vi "__Update Local List.vi"(8 "error in (no error)":errorcluster, 10 "Path to list":path, 11 "FileManager Ctl Refs in":T1) -> (0 "error out":errorcluster, 3 "FileManager Ctl Refs out":T1)   [LabVIEW 2011]
doc: "Lists the files and folders that reside under the specified path on the local system and updates the Local list with the items."
uses:
  __File manager Data type.ctl
  <vilib>/Utility/miscctls.llb/LVRowAndColumnUnsignedTypeDef.ctl
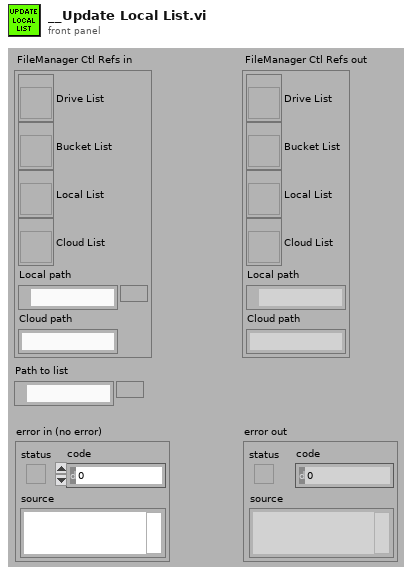
[diagram p1: front panel]
types:
  T1 = typedef "__File manager Data type.ctl" = cluster{"Drive List":refnum<vi>, "Bucket List":refnum<vi>, "Local List":refnum<vi>, "Cloud List":refnum<vi>, "Local path":path, "Cloud path":string}
  T2 = typedef "LVRowAndColumnUnsignedTypeDef.ctl" = cluster{"Row":u32, "Column":u32}
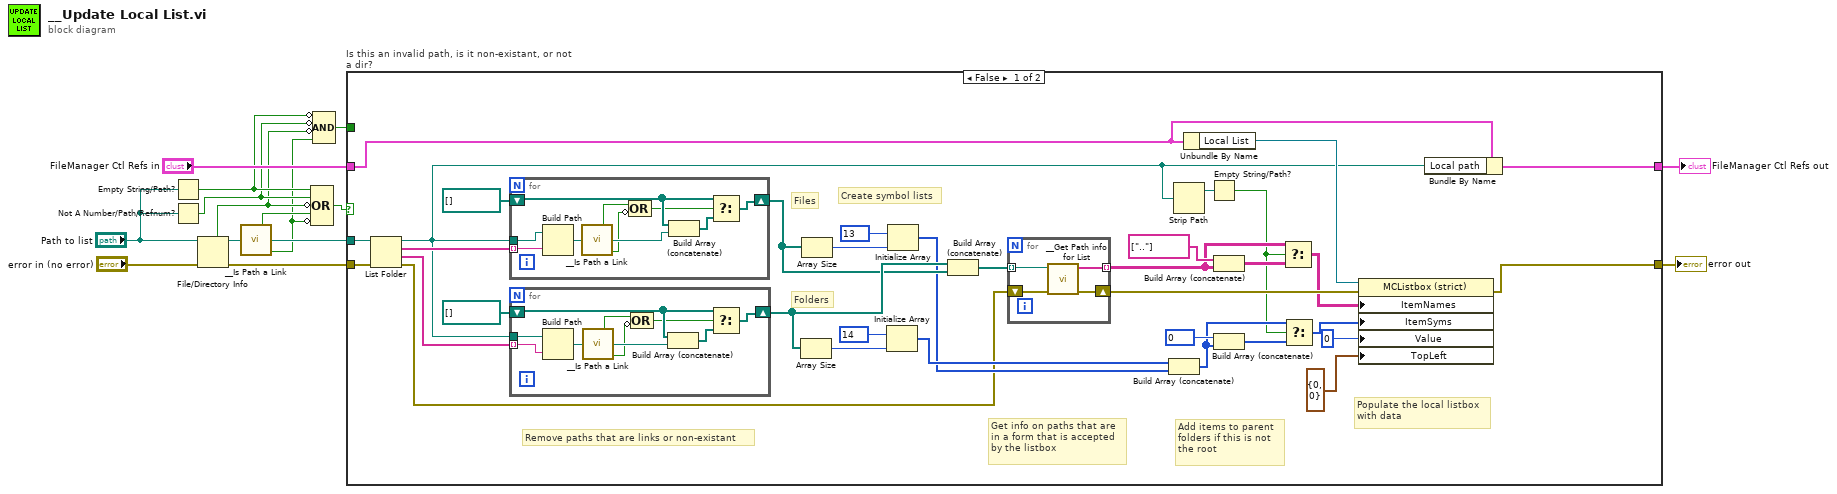
[diagram p0: block diagram]
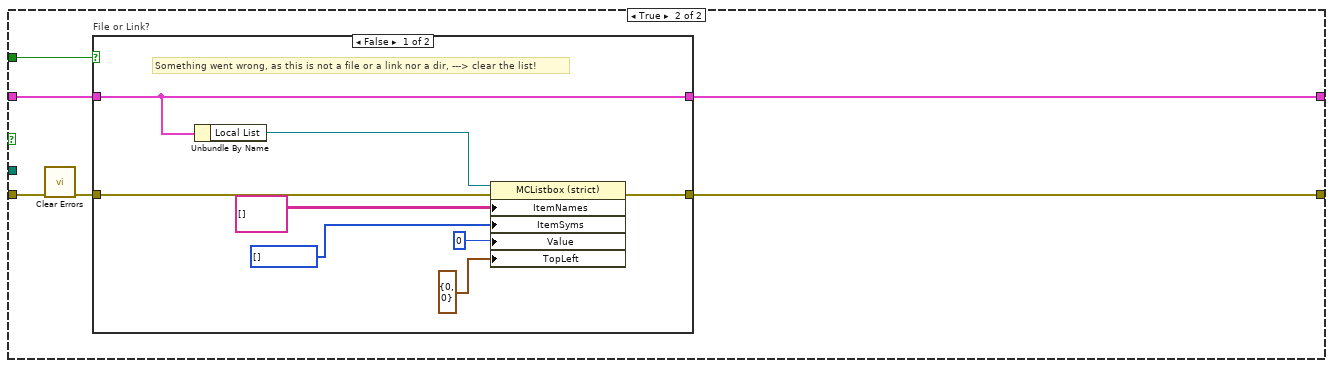
[diagram p2: hidden frame]
diagram:
  n1 = Empty String/Path?(string/path="Path to list") -> (empty?=w5:bool)
  n2 = Not A Number/Path/Refnum?(number/path/refnum="Path to list") -> (NaN/Path/Refnum?=w4:bool)
  n3 = File/Directory Info(path="Path to list", error in="error in (no error)") -> (path out=w11:path, directory=w3:bool, error out=w8:errorcluster)  [unwired: 4 out]
  n4 = call "__Is Path a Link.vi"("Path in"=w11) -> ("Link?"=w10:bool, "Path out"=w9:path, "Exists?"=w2:bool)  [unwired: 12 in]
  n5 = Compound Arithmetic op=OR(w5, w4, invert w3, w10, invert w2) -> (w12:bool)
  n6 = Compound Arithmetic op=AND(invert w5, invert w4, invert w3, w2) -> (w1:bool)
  n7 = case "Is this an invalid path, is it non-existant, or not a dir?" shown="False" w12 {
    tunnel: w8 -> [w16 w77]
    tunnel: [w49 w78] -> w15
    tunnel: "FileManager Ctl Refs in" -> [w48 w79]
    tunnel: [w47 w75] -> w13
    tunnel: w9 -> [w46 _]
    tunnel: w1 -> [_ w74]
    frame False {
      # "Add items to parent\nfolders if this is not\nthe root"
      # "Populate the local listbox\nwith data"
      # "Create symbol lists"
      # "Get info on paths that are\nin a form that is accepted\nby the listbox"
      # "Remove paths that are links or non-existant"
      # "Files"
      # "Folders"
      n8 = List Folder(path=w46, error in=w16) -> (path out=w27:path, filenames=w45:string[], folder names=w44:string[], error out=w31:errorcluster)  [unwired: 2 in]
      n9 = for {
        tunnel: w45 -> [w68] mode=indexing
        tunnel: w27 -> [w73]
        shift-right: [w71] -> w38
        shift-left: path[] [] -> [w69]
        n10 = Build Path(base path=w73, name or relative path=w68) -> (appended path=w72:path)
        n11 = call "__Is Path a Link.vi"("Path in"=w72) -> ("Link?"=w66:bool, "Path out"=w67:path, "Exists?"=w65:bool)  [unwired: 12 in]
        n12 = Compound Arithmetic op=OR(w66, invert w65) -> (w64:bool)
        n13 = Build Array (concatenate)(w69, w67) -> (w70:path[])
        n14 = Select(t=w69, s=w64, f=w70) -> (s? t:f=w71:path[])
      }
      n15 = for {
        tunnel: w44 -> [w59] mode=indexing
        tunnel: w27 -> [w63]
        shift-right: [w61] -> w39
        shift-left: path[] [] -> [w57]
        n16 = Build Path(base path=w63, name or relative path=w59) -> (appended path=w62:path)
        n17 = call "__Is Path a Link.vi"("Path in"=w62) -> ("Link?"=w56:bool, "Path out"=w58:path, "Exists?"=w54:bool)  [unwired: 12 in]
        n18 = Compound Arithmetic op=OR(w56, invert w54) -> (w55:bool)
        n19 = Build Array (concatenate)(w57, w58) -> (w60:path[])
        n20 = Select(t=w57, s=w55, f=w60) -> (s? t:f=w61:path[])
      }
      n21 = Array Size(array=w39) -> (size(s)=w40:i32)
      n22 = Array Size(array=w38) -> (size(s)=w43:i32)
      n23 = Initialize Array(14, w40) -> (w37:i32[])
      n24 = Initialize Array(13, w43) -> (w36:i32[])
      n25 = Build Array (concatenate)(w39, w38) -> (w34:path[])
      n26 = for {
        tunnel: w34 -> [w53] mode=indexing
        shift-right: [w51] -> w29
        shift-left: w31 -> [w52]
        tunnel: [w50] -> w25 mode=indexing
        n27 = call "__Get Path info for List.vi"("error in (no error)"=w52, "Path in"=w53) -> ("error out"=w51:errorcluster, "Path info"=w50:string[])  [unwired: 8 in]
      }
      n28 = Build Array (concatenate)(w37, w36) -> (w21:i32[])
      n29 = Strip Path(path=w27) -> (stripped path=w26:path)  [unwired: 1 out]
      n30 = Unbundle By Name(w48) -> ("Local List"=w28:refnum<vi>)
      n31 = Empty String/Path?(string/path=w26) -> (empty?=w20:bool)
      n32 = Build Array (concatenate)(string[] [".."], w25) -> (w24:string[][])
      n33 = Build Array (concatenate)(0, w21) -> (w22:i32[])
      n34 = Select(t=w25, s=w20, f=w24) -> (s? t:f=w23:string[][])
      n35 = Select(t=w21, s=w20, f=w22) -> (s? t:f=w19:i32[])
      n36 = property class="MCListbox (strict)"(reference=w28, error in=w29, "ItemNames"=w23, "ItemSyms"=w19, "Value"=0, "TopLeft"=T2 {"Row"=0, "Column"=0} ("Top Left Visible Cell")) -> (error out=w49:errorcluster)  [unwired: 1 out]
      n37 = Bundle By Name(cluster=w48, "Local path"=w27) -> (w47:T1)
    }
    frame True {
      n38 = call <vilib>:"Clear Errors.vi"("error in (no error)"=w77) -> ("error out"=w76:errorcluster)  [unwired: 6 in]
      n39 = case "File or Link?" shown="False" w74 {
        tunnel: w79 -> [w80 w89]
        tunnel: [w85 w88] -> w78
        tunnel: w76 -> [w81 w88]
        tunnel: [w80 w89] -> w75
        frame False {
          # "Something went wrong, as this is not a file or a link nor a dir, ---> clear the list!"
          n40 = Unbundle By Name(w80) -> ("Local List"=w84:refnum<vi>)
          n41 = property class="MCListbox (strict)"(reference=w84, error in=w81, "ItemNames"=string[][] [], "ItemSyms"=i32[] [], "Value"=0, "TopLeft"=T2 {"Row"=0, "Column"=0} ("Top Left Visible Cell")) -> (error out=w85:errorcluster)  [unwired: 1 out]
        }
        frame True {
        }
      }
    }
  }
  "FileManager Ctl Refs out" <- w13
  "error out" <- w15
